vi "Global Var.vi"() -> ()   [LabVIEW 2021, in "NMEA_GPS Ublox M8N.lvlib"]
uses:
  NMEA_GPS Ublox M8N.lvlib
panel:
  out "Exit GPS":bool
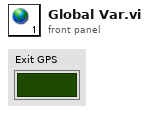
[diagram p1: front panel]
diagram:
